vi "Time To String.vi"(11 "Time":timestamp) -> (3 "date/time string":string)   [LabVIEW 2020, in "DataBase.lvlib"]
uses:
  DataBase.lvlib
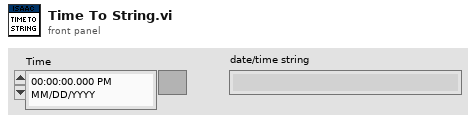
[diagram p1: front panel]
types:
  T1 = typedef "LVDateTimeRec.ctl" = cluster{"fractional second":dbl, "second":i32, "minute":i32, "hour":i32, "day of month":i32, "month":i32, "year":i32, "day of week":i32, "day of year":i32, "DST":i32}
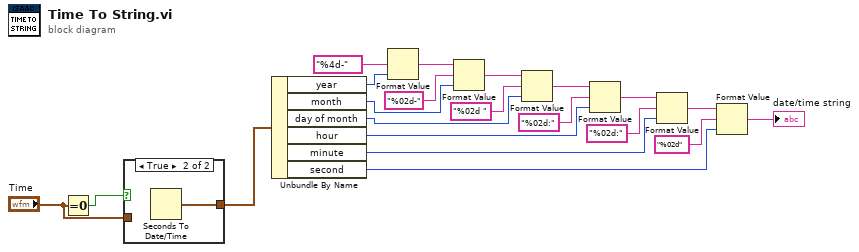
[diagram p0: block diagram]
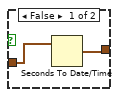
[diagram p2: hidden frame]
diagram:
  n1 = Equal To 0?(x="Time") -> (x = 0?=w21:bool)
  n2 = case shown="True" w21 {
    tunnel: [w22 w24] -> w20
    tunnel: "Time" -> [w23 _]
    frame False {
      n3 = Seconds To Date/Time(time stamp (now)=w23) -> (date time rec=w22:T1)  [unwired: 1 in]
    }
    frame True {
      n4 = Seconds To Date/Time() -> (date time rec=w24:T1)  [unwired: 2 in]
    }
  }
  n5 = Unbundle By Name(w20) -> ("year"=w15:i32, "month"=w16:i32, "day of month"=w17:i32, "hour"=w3:i32, "minute"=w6:i32, "second"=w7:i32)
  n6 = Format Value(format string="%4d-", value (0)=w15) -> (output string=w12:string)  [unwired: 1 in]
  n7 = Format Value(string ("")=w12, format string="%02d-", value (0)=w16) -> (output string=w13:string)
  n8 = Format Value(string ("")=w13, format string="%02d ", value (0)=w17) -> (output string=w14:string)
  n9 = Format Value(string ("")=w14, format string="%02d:", value (0)=w3) -> (output string=w4:string)
  n10 = Format Value(string ("")=w4, format string="%02d:", value (0)=w6) -> (output string=w5:string)
  n11 = Format Value(string ("")=w5, format string="%02d", value (0)=w7) -> (output string=→"date/time string":string)
